vi "Status SpecimenTempInfo.vi"(8 "error in (no error)":errorcluster, 10 "Address (0)":i32, 11 "VISA resource name":refnum<visa-resource-name>) -> (0 "error out":errorcluster, 1 "equipped with control function":bool, 2 "equipped with monitor function":bool, 3 "VISA resource name out":refnum<visa-resource-name>)   [LabVIEW 2016, in "Environment Chamber.lvlib" / "Climatic Chamber.lvlib"]
doc: "<B>On-board specimen temperature information monitor\n(P-200, P-300 controllers only)</B>\n\nReturns information about the on-board specimen temperature equipment."
uses:
  Climatic Chamber.lvlib
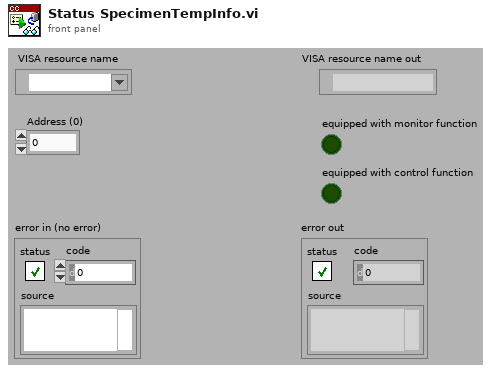
[diagram p1: front panel]
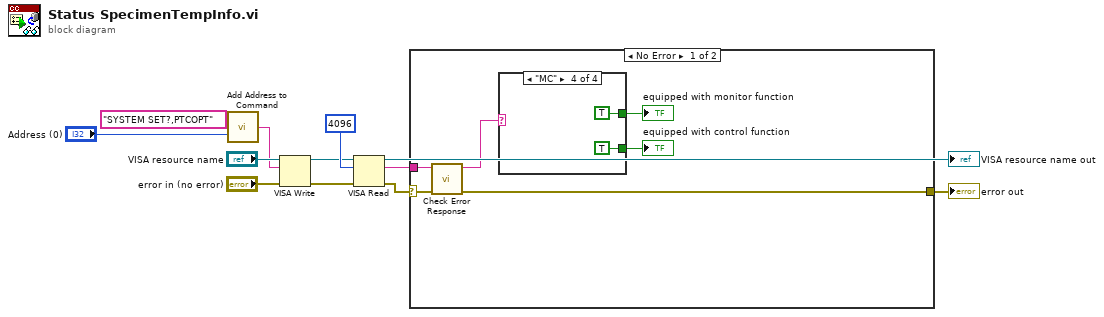
[diagram p0: block diagram]
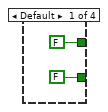
[diagram p2: hidden frame]
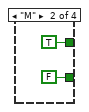
[diagram p3: hidden frame]
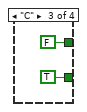
[diagram p4: hidden frame]
diagram:
  n1 = call "Add Address to Command.vi"("Address (0)"="Address (0)", "Command"="SYSTEM SET?,PTCOPT") -> ("Command OUT"=w5:string)
  n2 = VISA Write(VISA resource name="VISA resource name", write buffer=w5, error in (no error)="error in (no error)") -> (VISA resource name out=w9:refnum<visa-resource-name>, error out=w8:errorcluster)  [unwired: 1 out]
  n3 = VISA Read(VISA resource name=w9, byte count=u32 4096, error in (no error)=w8) -> (VISA resource name out=→"VISA resource name out":refnum<visa-resource-name>, read buffer=w3:string, error out=w4:errorcluster)  [unwired: 1 out]
  n4 = case shown="No Error" w4 {
    selector: w4 -> [w17 w27]
    tunnel: w3 -> [w18 _]
    tunnel: [w16 w27] -> w2
    frame No Error {
      n5 = call "Check Error Response.vi"("error in (no error)"=w17, "read String"=w18) -> ("error out"=w16:errorcluster, "String out"=w15:string)  [unwired: 7 in, 1 out]
      n6 = case shown="\"MC\"" w15 {
        tunnel: [FALSE TRUE FALSE TRUE] -> w13
        tunnel: [FALSE FALSE TRUE TRUE] -> w14
        frame Default {
        }
        frame "M" {
        }
        frame "C" {
        }
        frame "MC" {
        }
      }
      "equipped with control function" <- w14
      "equipped with monitor function" <- w13
    }
    frame Error {
    }
  }
  "error out" <- w2
